vi "Get Slaves.vi"(8 "error in (no error)":errorcluster, 11 "EtherCAT Master in":T3 {"VS ref" format="%.0x"}) -> (0 "error out":errorcluster, 1 "ECAT Generic Slaves":T2(array[cluster]) {"VS ref" format="%.0x"}, 2 "ECAT Slaves":T2(array[cluster]) {"VS ref" format="%.0x"}, 3 "EtherCAT Master out":T3 {"VS ref" format="%.0x"}, 4 "ECAT REM Slaves":T2(array[cluster]) {"VS ref" format="%.0x"})   [LabVIEW 2016, in "Scan Engine Custom Device.lvlib"]
uses:
  Scan Engine Custom Device.lvlib
  <vilib>/NI Veristand/Custom Device API/Custom Device API.lvlib
  Globals/Scan Engine GUIDs.vi
  <vilib>/NI Veristand/Custom Device API/Custom Device Item Ref.ctl
  <resource>/objmgr/IndComECAT.rc
  <vilib>/NI Veristand/Custom Device Tools/Custom Device Utility Library/Custom Device Utility Library.lvlib
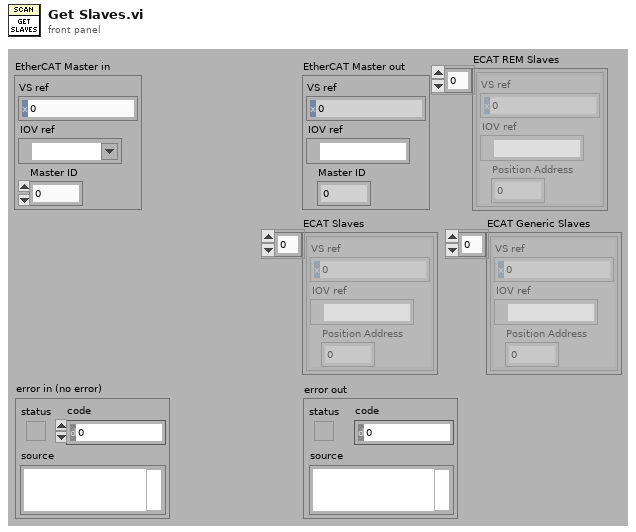
[diagram p1: front panel]
types:
  T1 = typedef "Custom Device API.lvlib/Custom Device Item Ref.ctl" = u64
  T2 = cluster{"VS ref":T1, "IOV ref":refnum<k21>, "Position Address":u16}[]
  T3 = cluster{"VS ref":T1, "IOV ref":refnum<k21>, "Master ID":u32}
  T4 = cluster{"ECAT Slave refs":T1[], "All ECAT Slaves":refnum<k21>[]}
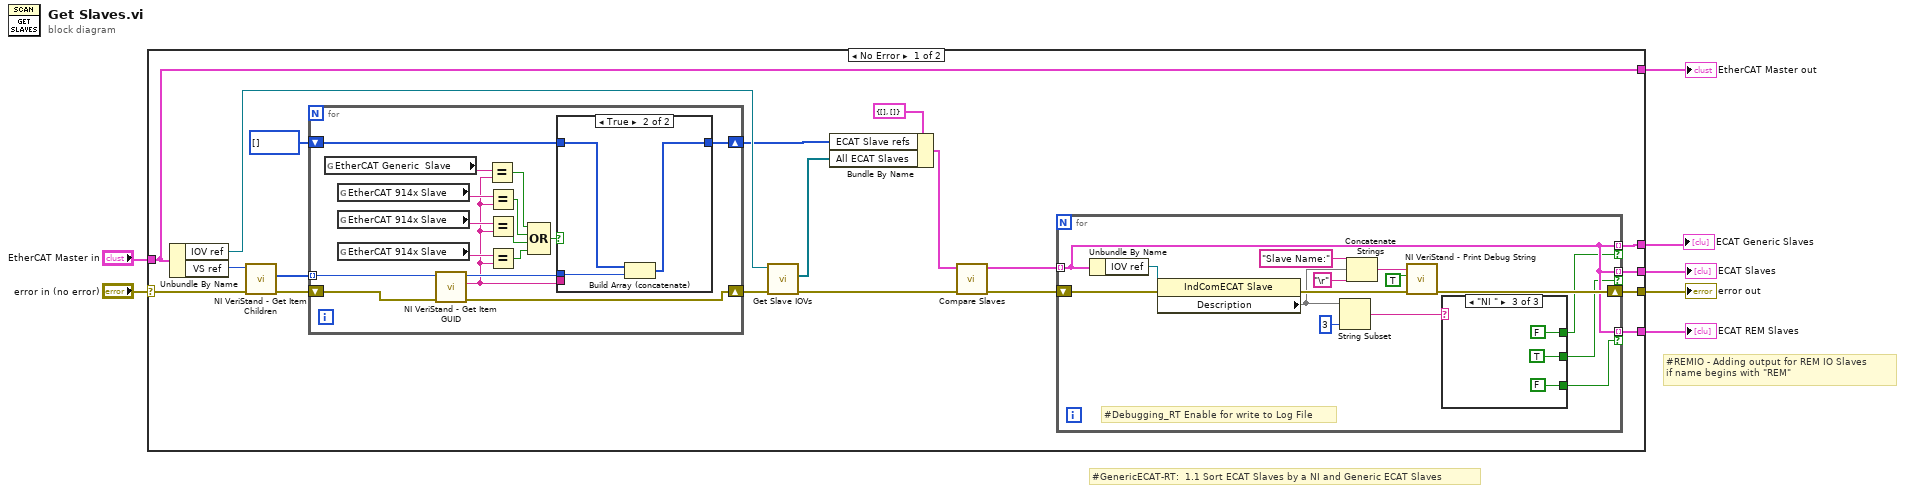
[diagram p0: block diagram]
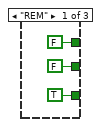
[diagram p2: hidden frame]
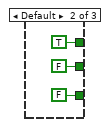
[diagram p3: hidden frame]
diagram:
  # "#REMIO - Adding output for REM IO Slaves\nif name begins with \"REM\""
  # "#GenericECAT-RT:  1.1 Sort ECAT Slaves by a NI and Generic ECAT Slaves"
  n1 = case shown="No Error" "error in (no error)" {
    selector: "error in (no error)" -> [w23 w72]
    tunnel: [w10 w72] -> w7
    tunnel: [w16 w71] -> w4
    tunnel: "EtherCAT Master in" -> [w16 w71]
    tunnel: [w12 _] -> w3
    tunnel: [w11 _] -> w2
    tunnel: [w8 _] -> w1
    frame No Error {
      n2 = Unbundle By Name(w16) -> ("IOV ref"=w18:refnum<k21>, "VS ref"=w19:T1)
      n3 = call <vilib>:"NI VeriStand - Get Item Children.vi"("error in (no error)"=w23, "Item Ref in"=w19) -> ("error out"=w24:errorcluster, "Child Refs"=w25:T1[])  [unwired: 6 in, 2 out]
      n4 = for {
        tunnel: w25 -> [w66] mode=indexing
        shift-right: [w62] -> w9
        shift-left: T1[] [] -> [w63]
        shift-right: [w60] -> w21
        shift-left: w24 -> [w61]
        n5 = global read "Scan Engine GUIDs.vi" "EtherCAT Generic  Slave"() -> (w58:string)
        n6 = global read "Scan Engine GUIDs.vi" "EtherCAT 914x Slave"() -> (w56:string)
        n7 = global read "Scan Engine GUIDs.vi" "EtherCAT 914x Slave"() -> (w57:string)
        n8 = global read "Scan Engine GUIDs.vi" "EtherCAT 914x Slave"() -> (w65:string)
        n9 = call <vilib>:"NI VeriStand - Get Item GUID.vi"("error in (no error)"=w61, "Item Ref in"=w66) -> ("error out"=w60:errorcluster, "GUID"=w53:string, "Item Ref out"=w64:T1)  [unwired: 7 in]
        n10 = Equal?(x=w58, y=w53) -> (x = y?=w55:bool)
        n11 = Equal?(x=w56, y=w53) -> (x = y?=w51:bool)
        n12 = Equal?(x=w57, y=w53) -> (x = y?=w52:bool)
        n13 = Equal?(x=w65, y=w53) -> (x = y?=w54:bool)
        n14 = Compound Arithmetic op=OR(w55, w51, w52, w54) -> (w59:bool)
        n15 = case shown="True" w59 {
          tunnel: w64 -> [_ w69]
          tunnel: w63 -> [w67 w70]
          tunnel: [w67 w68] -> w62
          tunnel: w53 -> [_ _]
          frame False {
          }
          frame True {
            n16 = Build Array (concatenate)(w70, w69) -> (w68:T1[])
          }
        }
      }
      n17 = call "Get Slave IOVs.vi"("error in (no error)"=w21, "ECAT Master in"=w18) -> ("error IO"=w15:errorcluster, "All Slaves"=w20:refnum<k21>[])  [unwired: 7 in, 1 out]
      n18 = Bundle By Name(cluster=T4 {"ECAT Slave refs"=[], "All ECAT Slaves"=[]} ("ECAT Slaves"), "ECAT Slave refs"=w9, "All ECAT Slaves"=w20) -> (w17:T4)
      n19 = call "Compare Slaves.vi"("error in (no error)"=w15, "ECAT Slaves in"=w17) -> ("error out"=w13:errorcluster, "ECAT Slaves out"=w14:T2)  [unwired: 8 in]
      n20 = for {
        tunnel: w14 -> [w30] mode=indexing
        tunnel: [w30] -> w11 mode=indexing if=w29
        tunnel: [w30] -> w12 mode=indexing if=w28
        shift-right: [w36] -> w10
        shift-left: w13 -> [w40]
        tunnel: [w30] -> w8 mode=indexing if=w27
        # "#Debugging_RT Enable for write to Log File"
        n21 = Unbundle By Name(w30) -> ("IOV ref"=w41:refnum<k21>)
        n22 = property class="IndComECAT Slave"(reference=w41, error in=w40) -> (error out=w34:errorcluster, "Description"=w32)  [unwired: 1 out]
        n23 = String Subset(string=w32, length (rest)=3 ("Länge (Rest)")) -> (substring=w31:string)  [unwired: 1 in]
        n24 = Concatenate Strings("Slave Name:", w32, "\r") -> (w37:string)
        n25 = call <vilib>:"NI VeriStand - Print Debug String.vi"("error in (no error)"=w34, "Add to log file? (T)"=TRUE, "Message"=w37) -> ("error out"=w36:errorcluster)  [unwired: 8 in]
        n26 = case shown="\"NI \"" w31 {
          tunnel: [FALSE TRUE FALSE] -> w29
          tunnel: [FALSE FALSE TRUE] -> w28
          tunnel: [TRUE FALSE FALSE] -> w27
          frame "REM" {
          }
          frame Default {
          }
          frame "NI " {
          }
        }
      }
    }
    frame Error {
    }
  }
  "error out" <- w7
  "EtherCAT Master out" <- w4
  "ECAT Slaves" <- w3
  "ECAT Generic Slaves" <- w2
  "ECAT REM Slaves" <- w1
